vi "1_Boolean_Adder_Logistic_Regression(Train).vi"() -> ()   [LabVIEW 2020]
uses:
  <vilib>/Ngene/DeepLTK/Toolkit/NN_Train/Controls/NN_Train_Params.ctl
  <vilib>/Ngene/DeepLTK/Toolkit/NN_Train/Controls/NN_Train_Optimizer.ctl
  <vilib>/Ngene/DeepLTK/Toolkit/NN_Train/Controls/NN_Train_Data_Sampling.ctl
  <vilib>/Ngene/DeepLTK/Toolkit/NN_Train/Controls/NN_LR_Policy_Cfg.ctl
  <vilib>/Ngene/DeepLTK/Toolkit/NN_Train/Controls/NN_LR_Policy_Type.ctl
  <vilib>/Ngene/DeepLTK/Toolkit/NN_Train/Controls/NN_Train_Session_Data.ctl
  <vilib>/Ngene/DeepLTK/Toolkit/NN_Data/API/DataSet_Types/NN_DataSet(In1D_Out1D).ctl
  <vilib>/Ngene/DeepLTK/Toolkit/NN_Data/API/DataRef_Types/NN_Data_ref(2D_SGL).ctl
  <vilib>/Ngene/DeepLTK/Toolkit/NN_Data/API/DataRef_Types/NN_Data_ref(1D_I32).ctl
  <vilib>/Ngene/DeepLTK/Toolkit/NN_Layers/Layers/Input/Controls/NN_Layer_Config(Input1D).ctl
  <vilib>/Ngene/DeepLTK/Toolkit/NN_Layers/Layers/FC/Controls/NN_Layer_Config(FC).ctl
  <vilib>/Ngene/DeepLTK/Toolkit/NN_Activations/Controls/NN_Activation_Type.ctl
  <vilib>/Ngene/DeepLTK/Toolkit/NN_Layers/Controls/NN_Layer_Init_Params.ctl
  <vilib>/Ngene/DeepLTK/Toolkit/NN_Layers/Controls/NN_Layer_Weight_Init_Type.ctl
  <vilib>/Ngene/DeepLTK/Toolkit/NN_Network/Controls/NN_Save_Before_Destroy_Options.ctl
  <vilib>/Ngene/DeepLTK/Toolkit/NN_Network/Controls/NN_Device.ctl
  <vilib>/Ngene/DeepLTK/Toolkit/NN_Layers/Layers/Input/NN_Layer_Create(Input1D).vi
  <vilib>/Ngene/DeepLTK/Toolkit/NN_Layers/Layers/FC/NN_Layer_Create(FC).vi
  <vilib>/Ngene/DeepLTK/Toolkit/NN_Train/Loss_Functions/NN_Set_Loss(MSE).vi
  <vilib>/Ngene/DeepLTK/Toolkit/NN_Network/subVIs/NN_Predict/NN_Predict(In1D_Out1D).vi
  <vilib>/Ngene/DeepLTK/Toolkit/NN_Train/Eval_Loss/NN_Eval_Test_Error_Loss/NN_Eval(In1D_Out1D).vi
  <vilib>/Ngene/DeepLTK/Toolkit/Deep_Learning_Toolkit_by_Ngene.lvlib
panel:
  out "Error Rate":sgl format="%#_3p"
  out "Dataset_Size":i32=65536
  out "Dims_Out":i32=8
  out "Dims_In":i32=16
  out "Train Loss":sgl=0.012967891 format="%#_4p"
  in  "Eval?":bool
  out "Session Data":T1={"Epochs"=17.482422, "Tot_Iter"=8951, "LR"=0.005, "LR_iter"=8952}
  in  "LR_Decay_Params":T2={"Policy_Type"=enum."Step", "LR0"=0.009999999999999998, "k"=10.0, "WarmUp_Policy"=enum."Ramp", "WarmUp_Iter"=1000, "WarmUp_Ratio"=10.0} {"WarmUp_Ratio" min=1; "WarmUp_Iter" min=1; "LR0" format="%.7f"}
  in  "?":bool
  out "Graphs":cluster{"Loss":sgl, "Error":sgl}(graph)={"Loss"=0.012967891, "Error"=0.0}
  in  "NN_Train_Params":T4={"Optimizer"=enum."Adam", "Beta_1"=0.9, "Beta_2"=0.999, "Weight Decay(L1)"=1e-08, "Weight Decay(L2)"=1e-08, "Data_Sampling"=enum."Random"}
  # "Overview: Demonstrates the usage of DeepLTK (Deep Learning Toolkit for LabVIEW) for solving a 8-bt Boolean Adder problem.\nRequirements: DeepLTK - Deep Learning Toolkit for LabVIEW (https://www.ngene.co/deep-learning-toolkit-for-labview)\nInstructions:\n1. Run the VI with default configurations.\n2. Observe how the training loss is decreasing.\n3. Periodically press \"Eval?\" button to observe \"Error Rate\" (relative number of incorrectly predicted samples).\n4. Press \"Stop\" when \"Error Rate\" is reaches 0. It should take 10-30 epochs to train.\nMore Examples:  https://github.com/ngenehub/deepltk_examples"
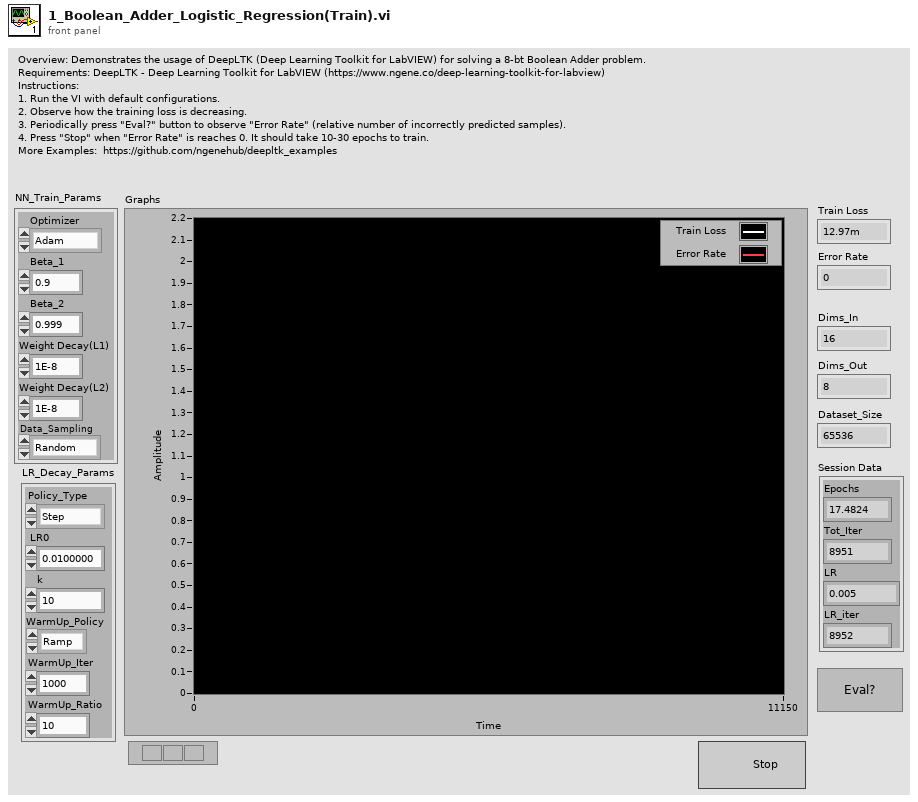
[diagram p1: front panel]
types:
  T1 = typedef "Deep_Learning_Toolkit_by_Ngene.lvlib/NN_Train_Session_Data.ctl" = cluster{"Epochs":sgl, "Tot_Iter":i32, "LR":sgl, "LR_iter":i32}
  T2 = typedef "Deep_Learning_Toolkit_by_Ngene.lvlib/NN_LR_Policy_Cfg.ctl" = cluster{"Policy_Type":T3, "LR0":dbl, "k":sgl, "WarmUp_Policy":enum16{"Step", "Ramp"}, "WarmUp_Iter":i32, "WarmUp_Ratio":sgl}
  T3 = typedef "Deep_Learning_Toolkit_by_Ngene.lvlib/NN_LR_Policy_Type.ctl" = enum16{"Manual", "Step", "Exp", "1/t"}
  T4 = typedef "Deep_Learning_Toolkit_by_Ngene.lvlib/NN_Train_Params.ctl" = cluster{"Optimizer":T5, "Beta_1":sgl, "Beta_2":sgl, "Weight Decay(L1)":sgl, "Weight Decay(L2)":sgl, "Data_Sampling":T6}
  T5 = typedef "Deep_Learning_Toolkit_by_Ngene.lvlib/NN_Train_Optimizer.ctl" = enum16{"SGD", "Adam", "Adagrad", "Adadelta", "RMSProp", "Nesterov"}
  T6 = typedef "Deep_Learning_Toolkit_by_Ngene.lvlib/NN_Train_Data_Sampling.ctl" = enum16{"Random", "Sequential"}
  T7 = typedef "Deep_Learning_Toolkit_by_Ngene.lvlib/NN_Layer_Config(FC).ctl" = cluster{"Name":string, "Size":i32, "BN":bool, "Activation":T8, "Init_Params":T9, "Custom_Params":string}
  T8 = typedef "Deep_Learning_Toolkit_by_Ngene.lvlib/NN_Activation_Type.ctl" = enum16{"Sigmoid", "ReLU", "LReLU", "ReLU6", "tanh", "Swish", "Mish", "None"}
  T9 = typedef "Deep_Learning_Toolkit_by_Ngene.lvlib/NN_Layer_Init_Params.ctl" = cluster{"Init_Type":T10, "Value":sgl}
  T10 = typedef "Deep_Learning_Toolkit_by_Ngene.lvlib/NN_Layer_Weight_Init_Type.ctl" = enum16{"Const", "Uniform", "Gaussian", "Xavier"}
  T11 = typedef "Deep_Learning_Toolkit_by_Ngene.lvlib/NN_Device.ctl" = enum16{"CPU", "GPU"}
  T12 = typedef "Deep_Learning_Toolkit_by_Ngene.lvlib/NN_Save_Before_Destroy_Options.ctl" = cluster{"CFG?":bool, "Weights?":bool, "Render?":bool}
  T13 = typedef "Deep_Learning_Toolkit_by_Ngene.lvlib/NN_Layer_Config(Input1D).ctl" = cluster{"Name":string, "Size":i32}
  T14 = typedef "Deep_Learning_Toolkit_by_Ngene.lvlib/NN_DataSet(In1D_Out1D).ctl" = cluster{"Inputs Ref.":T15, "Outputs Ref.":T15, "Dims_In":i32, "Dataset_Size":i32, "Outputs_idx Ref.":T16, "Dims_Out":i32, "Labels":string[], "File Paths":path[]}
  T15 = typedef "Deep_Learning_Toolkit_by_Ngene.lvlib/NN_Data_ref(2D_SGL).ctl" = refnum<data-value>
  T16 = typedef "Deep_Learning_Toolkit_by_Ngene.lvlib/NN_Data_ref(1D_I32).ctl" = refnum<data-value>
  T17 = typedef "Deep_Learning_Toolkit_by_Ngene.lvlib/NN.ctl" = cluster{"Name":string, "No of Layers":i32, "mBatch":i32, "Layers":T18[], "Dimty":T19, "Dims_In":T20, "Dims_Out":T20, "Working_Dir":path, "Train?":bool, "Train_Params":T4, "LR_Update_Policy":T2, "Session Data":T1, "Ground_truth":T21, "NNg_hdls":T22, "NN_Device":T11, "GPU Id":i32, "Labels":string[], "Receptive Field":T23[], "Loss_Type":T24, "Loss_Cfg_Prms":variant}
  T18 = typedef "Deep_Learning_Toolkit_by_Ngene.lvlib/NN_Layer_ref.ctl" = refnum<data-value>
  T19 = typedef "Deep_Learning_Toolkit_by_Ngene.lvlib/NN_In_Out_Dim-ty.ctl" = enum8{"In1D_Out1D", "In3D_Out1D", "In3D_Out3D", "In3D_OutBBox"}
  T20 = typedef "Deep_Learning_Toolkit_by_Ngene.lvlib/NN_Dims(C,H,W).ctl" = cluster{"C":i32, "H":i32, "W":i32}
  T21 = typedef "Deep_Learning_Toolkit_by_Ngene.lvlib/NN_Ground_truth.ctl" = cluster{"Y":variant, "Y_idx":T16}
  T22 = typedef "Deep_Learning_Toolkit_by_Ngene.lvlib/nng_cuda_handles.ctl" = cluster{"cudnn":u64, "cublas":u64, "stream":u64, "curand":u64}
  T23 = typedef "Deep_Learning_Toolkit_by_Ngene.lvlib/NN_Dims(V,H).ctl" = cluster{"V":i32, "H":i32}
  T24 = typedef "Deep_Learning_Toolkit_by_Ngene.lvlib/NN_Loss_Type.ctl" = enum16{"None", "MSE", "CrossEntropy", "YOLO_v2"}
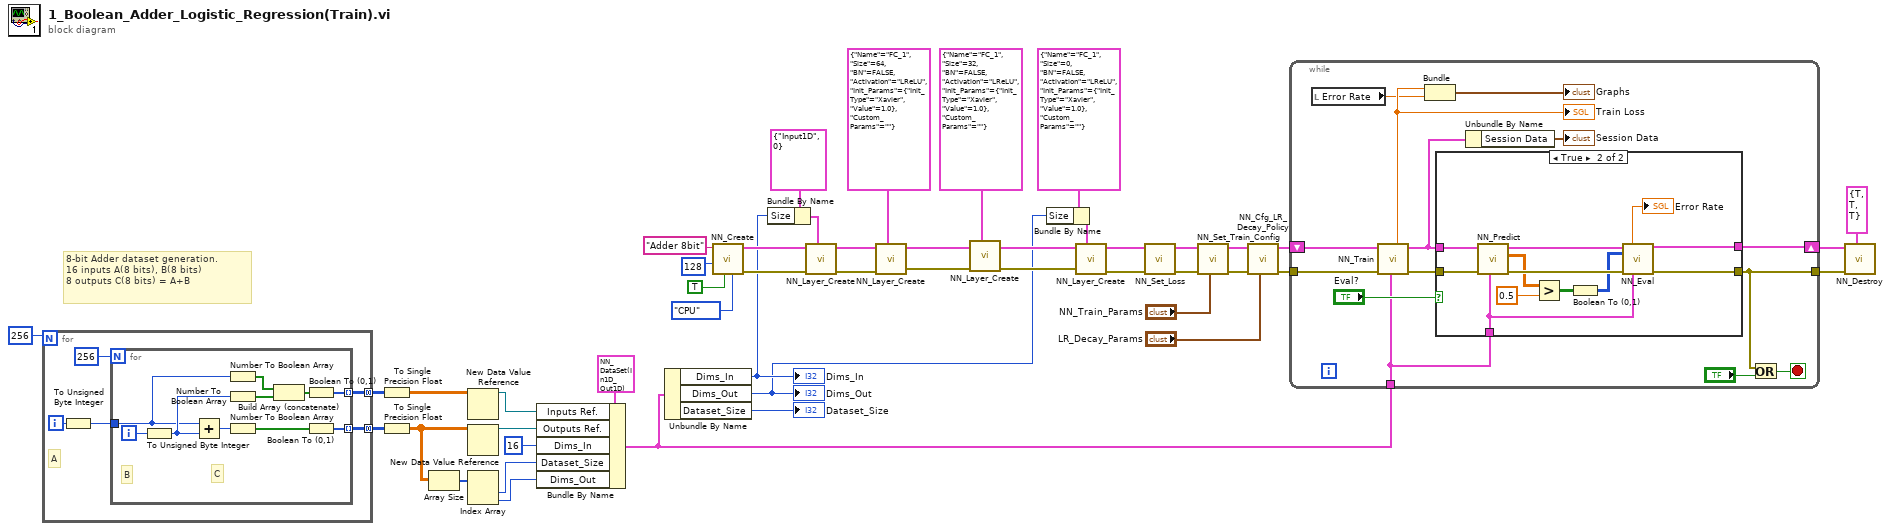
[diagram p0: block diagram]
diagram:
  # "8-bit Adder dataset generation.\n16 inputs A(8 bits), B(8 bits)\n8 outputs C(8 bits) = A+B"
  n1 = for {
    N: 256 -> [_]
    tunnel: [w51] -> w21 mode=concatenating
    tunnel: [w50] -> w20 mode=concatenating
    i -> [w49]
    # "A"
    n2 = To Unsigned Byte Integer(number=w49) -> (unsigned 8bit integer=w48:u8)
    n3 = for {
      N: 256 -> [_]
      tunnel: [w61] -> w50 mode=indexing
      tunnel: [w58] -> w51 mode=indexing
      tunnel: w48 -> [w55]
      i -> [w57]
      # "C"
      # "B"
      n4 = To Unsigned Byte Integer(number=w57) -> (unsigned 8bit integer=w56:u8)
      n5 = Add(x=w55, y=w56) -> (x+y=w59:u8)
      n6 = Number To Boolean Array(number=w55) -> (Boolean array=w53:bool[])
      n7 = Number To Boolean Array(number=w56) -> (Boolean array=w62:bool[])
      n8 = Number To Boolean Array(number=w59) -> (Boolean array=w60:bool[])
      n9 = Build Array (concatenate)(w53, w62) -> (w54:bool[])
      n10 = Boolean To (0,1)(Boolean=w54) -> (0, 1=w61:i16[])
      n11 = Boolean To (0,1)(Boolean=w60) -> (0, 1=w58:i16[])
    }
  }
  n12 = To Single Precision Float(number=w20) -> (single precision float=w6:sgl[][])
  n13 = To Single Precision Float(number=w21) -> (single precision float=w12:sgl[][])
  n14 = Array Size(array=w12) -> (size(s)=w11:i32[])
  n15 = New Data Value Reference(data value=w6) -> (data value reference=w46:refnum<data-value>)  [unwired: 1 in, 1 out]
  n16 = New Data Value Reference(data value=w12) -> (data value reference=w45:refnum<data-value>)  [unwired: 1 in, 1 out]
  n17 = Index Array(array=w11) -> (element #1=w10:i32, element #2=w8:i32)  [unwired: 2 in]
  n18 = Bundle By Name(cluster=T14 {"Inputs Ref."=refnum, "Outputs Ref."=refnum, "Dims_In"=0, "Dataset_Size"=0, "Outputs_idx Ref."=refnum, "Dims_Out"=0, "Labels"=[], "File Paths"=[]} ("Dataset(In1D_Out1D)"), "Inputs Ref."=w46, "Outputs Ref."=w45, "Dims_In"=16, "Dataset_Size"=w10, "Dims_Out"=w8) -> (w3:T14)
  n19 = Unbundle By Name(w3) -> ("Dims_In"=w9:i32, "Dims_Out"=w4:i32, "Dataset_Size"=→"Dataset_Size":i32)
  "Dims_In" <- w9
  "Dims_Out" <- w4
  n20 = call <vilib>:"NN_Create.vi"("NN_Device"=NN_Device."CPU", "Train? (false)"=TRUE, "mBatch (1)"=128, "Name"="Adder 8bit") -> ("error out"=w41:errorcluster, "NN out"=w42:T17)  [unwired: 6 in]
  n21 = Bundle By Name(cluster=T13 {"Name"="Input1D", "Size"=0} ("Input1D_Cfg"), "Size"=w9) -> (w36:T13)
  n22 = call-poly <vilib>:"NN_Layer_Create.vi"("Input1D_Cfg"=w36, "error in (no error)"=w41, "NN in"=w42) -> ("error out"=w44:errorcluster, "NN out"=w43:T17)  [unwired: 6 in, 1 out]
  n23 = call-poly <vilib>:"NN_Layer_Create.vi"("FC_Cfg"=T7 {"Name"="FC_1", "Size"=64, "BN"=FALSE, "Activation"=enum."LReLU", "Init_Params"={"Init_Type"=enum."Xavier", "Value"=1.0}, "Custom_Params"=""}, "error in (no error)"=w44, "NN in"=w43) -> ("error out"=w16:errorcluster, "NN out"=w17:T17)  [unwired: 6 in, 1 out]
  n24 = call-poly <vilib>:"NN_Layer_Create.vi"("FC_Cfg"=T7 {"Name"="FC_1", "Size"=32, "BN"=FALSE, "Activation"=enum."LReLU", "Init_Params"={"Init_Type"=enum."Xavier", "Value"=1.0}, "Custom_Params"=""}, "error in (no error)"=w16, "NN in"=w17) -> ("error out"=w15:errorcluster, "NN out"=w14:T17)  [unwired: 6 in, 1 out]
  n25 = Bundle By Name(cluster=T7 {"Name"="FC_1", "Size"=0, "BN"=FALSE, "Activation"=enum."LReLU", "Init_Params"={"Init_Type"=enum."Xavier", "Value"=1.0}, "Custom_Params"=""} ("FC_Cfg"), "Size"=w4) -> (w5:T7)
  n26 = call-poly <vilib>:"NN_Layer_Create.vi"("FC_Cfg"=w5, "error in (no error)"=w15, "NN in"=w14) -> ("error out"=w19:errorcluster, "NN out"=w18:T17)  [unwired: 6 in, 1 out]
  n27 = call-poly <vilib>:"NN_Set_Loss.vi"("error in (no error)"=w19, "NN in"=w18) -> ("error out"=w22:errorcluster, "NN out"=w23:T17)  [unwired: 8 in]
  n28 = call <vilib>:"NN_Set_Train_Config.vi"("NN_Train_Params"="NN_Train_Params", "error in (no error)"=w22, "NN in"=w23) -> ("error out"=w28:errorcluster, "NN out"=w33:T17)  [unwired: 7 in]
  n29 = call <vilib>:"NN_Cfg_LR_Decay_Policy.vi"("LR_Decay_Params"="LR_Decay_Params", "error in (no error)"=w28, "NN in"=w33) -> ("error out"=w27:errorcluster, "NN out"=w29:T17)  [unwired: 7 in]
  n30 = while {
    tunnel: w27 -> [w75]
    tunnel: w3 -> [w63]
    shift-right: [w69] -> w31
    shift-left: w29 -> [w76]
    tunnel: [w64] -> w30
    stop <- w73 stop-if-true
    n31 = local read "Error Rate"() -> (w65:sgl)
    n32 = call <vilib>:"NN_Train.vi"("Train Dataset"=w63, "error in (no error)"=w75, "NN in"=w76) -> ("error out"=w68:errorcluster, "NN out"=w71:T17, "Loss"=w72:sgl)  [unwired: 5 in, 1 out]
    "Train Loss" <- w72
    n33 = Bundle("Loss"=w72, "Error Rate"=w65) -> (→"Graphs":cluster{"Loss":sgl, "Error Rate":sgl})  [unwired: 1 in]
    n34 = case shown="True" "Eval?" {
      tunnel: w71 -> [w78 w85]
      tunnel: [w78 w90] -> w69
      tunnel: w68 -> [w77 w84]
      tunnel: [w77 w89] -> w64
      tunnel: w63 -> [_ w80]
      frame False {
      }
      frame True {
        n35 = call-poly <vilib>:"NN_Predict.vi"("Dataset"=w80, "error in (no error)"=w84, "NN in"=w85) -> ("error out"=w87:errorcluster, "Predictions"=w86:sgl[][], "NN out"=w88:T17)  [unwired: 6 in]
        n36 = Greater?(x=w86, y=sgl 0.5) -> (0:w83:bool[][])
        n37 = Boolean To (0,1)(Boolean=w83) -> (0, 1=w81:i16[][])
        n38 = call-poly <vilib>:"NN_Eval.vi"("NN in"=w88, "Predictions"=w81, "error in (no error)"=w87, "Dataset"=w80) -> ("Error"=→"Error Rate":sgl, "NN out"=w90:T17, "error out"=w89:errorcluster)  [unwired: 7 in, 2 out]
      }
    }
    n39 = Unbundle By Name(w71) -> ("Session Data"=→"Session Data":T1)
    n40 = Or(x=w64, y="?") -> (x .or. y?=w73:bool)
  }
  n41 = call <vilib>:"NN_Destroy.vi"("Save (T, T, T)"=T12 {"CFG?"=TRUE, "Weights?"=TRUE, "Render?"=TRUE}, "error in (no error)"=w30, "NN in"=w31) -> ()  [unwired: 8 in, 1 out]
